vi "SAC-Register Control Events.vi"(7 "Refs":refnum<vi>, 11 "error in (no error)":errorcluster) -> (4 "Event Registration Refnum":refnum<event-registration>, 15 "error out":errorcluster)   [LabVIEW 2020]
uses:
  SAC Config/Events.ctl
  SAC Config/Selection changed.ctl
  SAC Config/SAC Config.xctl
panel:
  in  "temp":cluster{"SAC Config":T1}
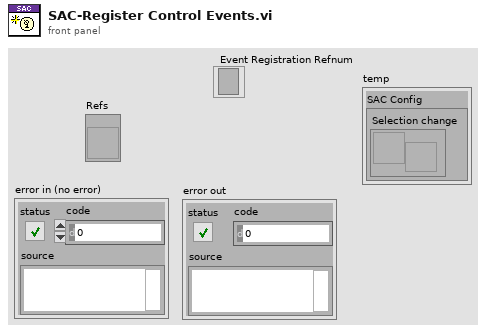
[diagram p1: front panel]
types:
  T1 = typedef "SAC Config.xctl/Events.ctl" = cluster{"Selection change":refnum<user-event>}
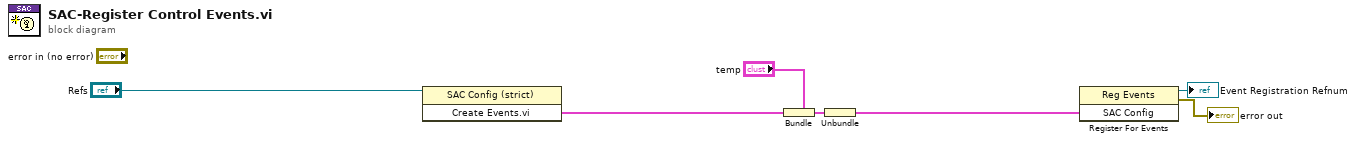
[diagram p0: block diagram]
diagram:
  n1 = invoke class="SAC Config (strict)" method="Create Events.vi"(reference="Refs") -> ("Create Events.vi"=w4:T1)  [unwired: 2 in, 2 out]
  n2 = Bundle(cluster="temp", "SAC Config"=w4) -> (w7:cluster{"SAC Config":T1})
  n3 = Unbundle(w7) -> ("SAC Config"=w3:T1)
  n4 = register-events(w3) -> (reference out=→"Event Registration Refnum":refnum<event-registration>, error out=→"error out":errorcluster)  [unwired: 2 in]
